vi "Read Commit Operation Errors.vi"(8 "Error In":errorcluster, 11 "Commit in":refnum<class "Commit.lvclass">) -> (0 "Error Out":errorcluster, 2 "Commit Operation Errors":errorcluster, 3 "Commit out":refnum<class "Commit.lvclass">)   [LabVIEW 2017, in "CL_G3_VIComponentBuilder.lvlib" / "Commit.lvclass"]
uses:
  Commit.lvclass
  Commit.lvclass/Commit.ctl
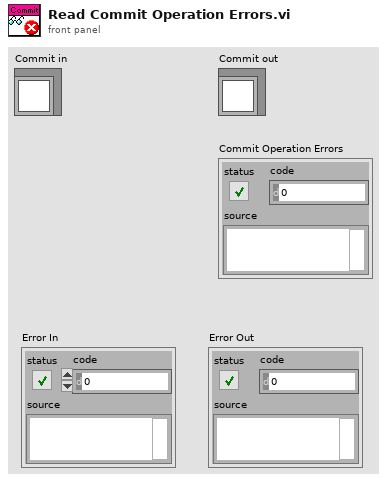
[diagram p1: front panel]
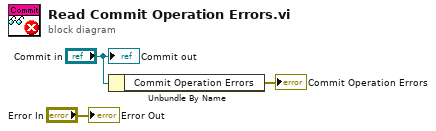
[diagram p0: block diagram]
diagram:
  n1 = Unbundle By Name("Commit in") -> ("Commit Operation Errors"=→"Commit Operation Errors":errorcluster)
  "Commit out" <- "Commit in"
  "Error Out" <- "Error In"
